vi "excel.vi"(4 "input cluster":T1, 5 "error out":errorcluster, 6 "fecha y hora":string, 7 "refnum out":refnum<file>, 8 "CH 4":dbl format="%#_13g", 9 "CH 3":dbl format="%#_13g", 10 "CH 2":dbl format="%#_13g", 11 "CH 1":dbl format="%#_13g") -> (2 "error in":errorcluster, 3 "refnum":refnum<file>)   [LabVIEW 2014]
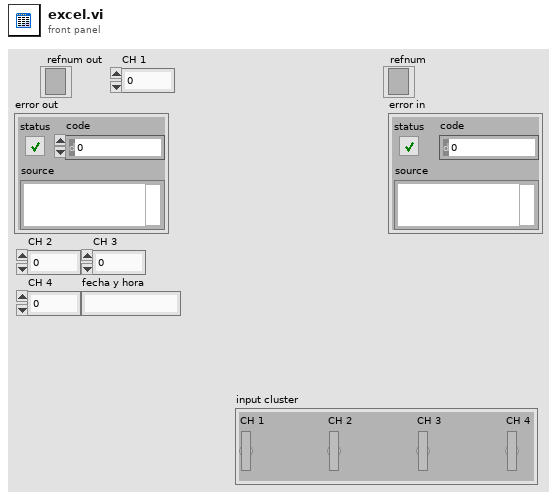
[diagram p1: front panel]
types:
  T1 = cluster{"CH 1":bool, "CH 2":bool, "CH 3":bool, "CH 4":bool}
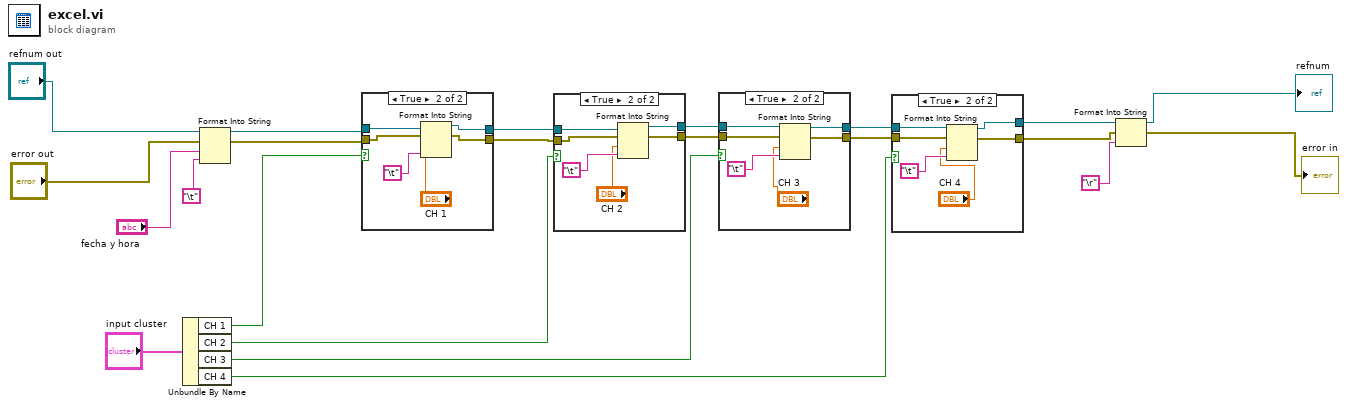
[diagram p0: block diagram]
diagram:
  n1 = Unbundle By Name("input cluster") -> ("CH 1"=w11:bool, "CH 2"=w10:bool, "CH 3"=w9:bool, "CH 4"=w8:bool)
  n2 = Format Into String(initial string="refnum out", error in="error out", "fecha y hora", "\t") -> (resulting string=w6:refnum<file>, error out=w5:errorcluster)  [unwired: 1 in]
  n3 = case shown="True" w11 {
    tunnel: w6 -> [w24 w30]
    tunnel: w5 -> [w23 w28]
    tunnel: [w24 w29] -> w22
    tunnel: [w23 w27] -> w21
    frame False {
    }
    frame True {
      n4 = Format Into String(initial string=w30, error in=w28, "CH 1", "\t") -> (resulting string=w29:refnum<file>, error out=w27:errorcluster)  [unwired: 1 in]
    }
  }
  n5 = case shown="True" w10 {
    tunnel: w22 -> [w32 w38]
    tunnel: w21 -> [w31 w35]
    tunnel: [w32 w37] -> w18
    tunnel: [w31 w36] -> w13
    frame False {
    }
    frame True {
      n6 = Format Into String(initial string=w38, error in=w35, "CH 2", "\t") -> (resulting string=w37:refnum<file>, error out=w36:errorcluster)  [unwired: 1 in]
    }
  }
  n7 = case shown="True" w9 {
    tunnel: w18 -> [w40 w46]
    tunnel: [w40 w45] -> w17
    tunnel: [w39 w44] -> w14
    tunnel: w13 -> [w39 w43]
    frame False {
    }
    frame True {
      n8 = Format Into String(initial string=w46, error in=w43, "CH 3", "\t") -> (resulting string=w45:refnum<file>, error out=w44:errorcluster)  [unwired: 1 in]
    }
  }
  n9 = case shown="True" w8 {
    tunnel: w17 -> [w48 w54]
    tunnel: [w48 w53] -> w16
    tunnel: [w47 w52] -> w15
    tunnel: w14 -> [w47 w51]
    frame False {
    }
    frame True {
      n10 = Format Into String(initial string=w54, error in=w51, "CH 4", "\t") -> (resulting string=w53:refnum<file>, error out=w52:errorcluster)  [unwired: 1 in]
    }
  }
  n11 = Format Into String(initial string=w16, error in=w15, "\r") -> (resulting string=→"refnum":refnum<file>, error out=→"error in":errorcluster)  [unwired: 1 in]
